vi "Calculate_Timescales.vi"(2 "Sampling Frequency (Hz)":dbl, 4 "Autocorrelation":dbl[](array[numeric])) -> (0 "Time between independent samples (s)":dbl, 1 "Timescale estimate (s)":dbl)   [LabVIEW 2016]
uses:
  <vilib>/Analysis/2dsp.llb/Integral Method.ctl
  <vilib>/Analysis/8numeric.llb/1D Numeric Integration.vi
  <vilib>/Analysis/NI_AALPro.lvlib
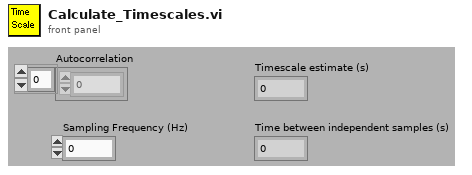
[diagram p1: front panel]
types:
  T1 = typedef "NI_AALPro.lvlib/Integral Method.ctl" = i32
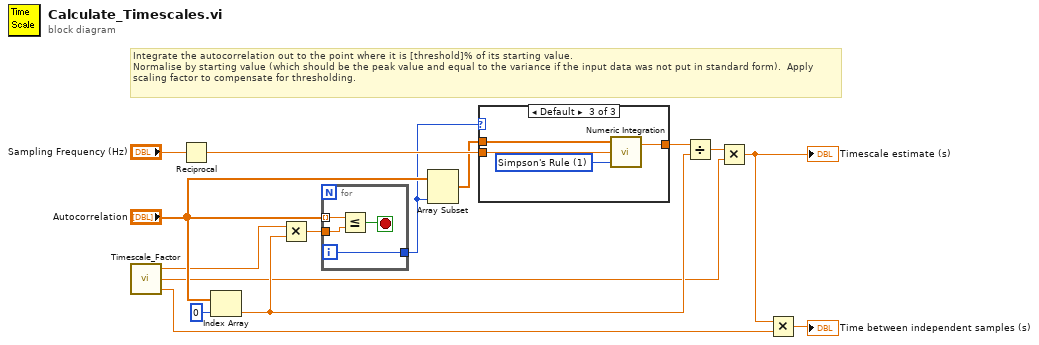
[diagram p0: block diagram]
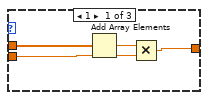
[diagram p2: hidden frame]
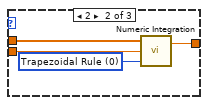
[diagram p3: hidden frame]
diagram:
  # "Integrate the autocorrelation out to the point where it is [threshold]% of its starting value.\nNormalise by starting value (which should be the peak value and equal to the variance if the input data was not put in standard form).  Apply scaling factor to compensate for thresholding."
  n1 = call "Timescale_Factor.vi"() -> ("Timescale multiplier for independent samples"=w6:dbl, "Timescale scaling factor"=w9:dbl, "Integration threshold (0...1)"=w10:dbl)  [unwired: 3 in]
  n2 = Reciprocal(x="Sampling Frequency (Hz)") -> (1/x=w3:dbl)
  n3 = Index Array(array="Autocorrelation", index=0) -> (element=w13:dbl)
  n4 = Multiply(x=w10, y=w13) -> (x*y=w12:dbl)
  n5 = for {
    tunnel: "Autocorrelation" -> [w17] mode=indexing
    tunnel: [w19] -> w1
    tunnel: w12 -> [w18]
    i -> [w19]
    stop <- w16 stop-if-true
    n6 = Less Or Equal?(x=w17, y=w18) -> (x <= y?=w16:bool)
  }
  n7 = Array Subset(array="Autocorrelation", length=w1) -> (w2:dbl[])  [unwired: 1 in]
  n8 = case shown="Default" w1 {
    tunnel: [w20 w26 w30] -> w4
    tunnel: w2 -> [w23 w25 w29]
    tunnel: w3 -> [w22 w24 w28]
    frame 1 {
      n9 = Add Array Elements(numeric array=w23) -> (sum=w21:dbl)
      n10 = Multiply(x=w21, y=w22) -> (x*y=w20:dbl)
    }
    frame 2 {
      w27 = T1 0 items=["Trapezoidal Rule", "Simpson's Rule", "Simpson's 3/8 Rule", "Bode Rule"] ("integration method")
      n11 = call-poly <vilib>:"Numeric Integration.vi"("integration method"=w27, "dt"=w24, "Input Array"=w25) -> ("result"=w26:dbl)  [unwired: 1 out]
    }
    frame Default {
      w31 = T1 1 items=["Trapezoidal Rule", "Simpson's Rule", "Simpson's 3/8 Rule", "Bode Rule"] ("integration method")
      n12 = call-poly <vilib>:"Numeric Integration.vi"("integration method"=w31, "dt"=w28, "Input Array"=w29) -> ("result"=w30:dbl)  [unwired: 1 out]
    }
  }
  n13 = Divide(x=w4, y=w13) -> (x/y=w8:dbl)
  n14 = Multiply(x=w8, y=w9) -> (x*y=w7:dbl)
  "Timescale estimate (s)" <- w7
  n15 = Multiply(x=w7, y=w6) -> (x*y=→"Time between independent samples (s)":dbl)
